vi "Save_Data_file_header_and_path_configuration.vi"(1 "Save":bool, 2 "path":path, 3 "File name":string="Name") -> (0 "Output Path":path)   [LabVIEW 2018]
uses:
  <vilib>/Utility/file.llb/Write To Spreadsheet File (string).vi
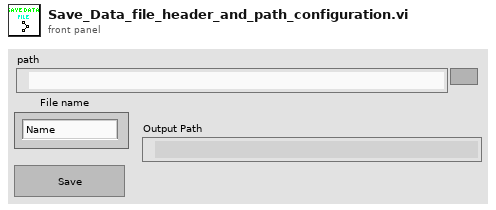
[diagram p1: front panel]
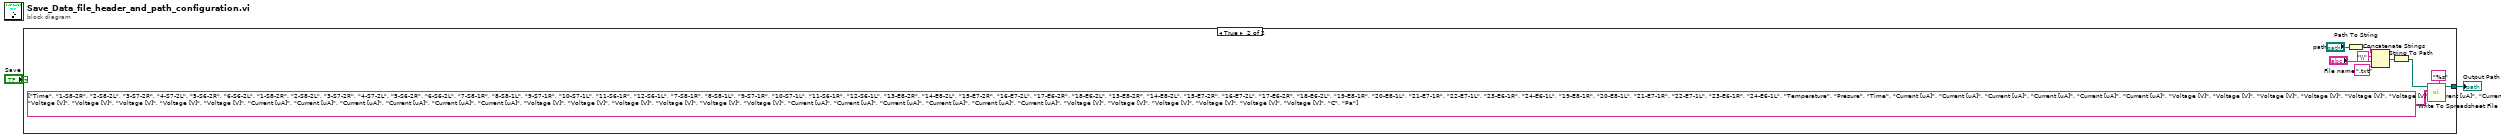
[diagram p0: block diagram]
diagram:
  n1 = case shown="True" "Save" {
    tunnel: [_ w6] -> w1
    frame False {
    }
    frame True {
      n2 = Path To String(path="path") -> (string=w5:string)
      n3 = Concatenate Strings(w5, "\\" ("string"), "File name", ".txt" ("string")) -> (w11:string)
      n4 = String To Path(string=w11) -> (path=w12:path)
      n5 = call-poly <vilib>:"Write To Spreadsheet File.vi"("format (%s)"="%s", "2D data"=string[][] [["Time", "1-S8-2R", "2-S8-2L", "3-S7-2R", "4-S7-2L", "5-S6-2R", "6-S6-2L", "1-S8-2R", "2-S8-2L", "3-S7-2R", "4-S7-2L", "5-S6-2R", "6-S6-2L", "7-S8-1R", "8-S8-1L", "9-S7-1R", "10-S7-1L", "11-S6-1R", "12-S6-1L", "7-S8-1R", "8-S8-1L", "9-S7-1R", "10-S7-1L", "11-S6-1R", "12-S6-1L", "13-E8-2R", "14-E8-2L", "15-E7-2R", "16-E7-2L", "17-E6-2R", "18-E6-2L", "13-E8-2R", "14-E8-2L", "15-E7-2R", "16-E7-2L", "17-E6-2R", "18-E6-2L", "19-E8-1R", "20-E8-1L", "21-E7-1R", "22-E7-1L", "23-E6-1R", "24-E6-1L", "19-E8-1R", "20-E8-1L", "21-E7-1R", "22-E7-1L", "23-E6-1R", "24-E6-1L", "Temperature", "Presure"], ["Time", "Current [uA]", "Current [uA]", "Current [uA]", "Current [uA]", "Current [uA]", "Current [uA]", "Voltage [V]", "Voltage [V]", "Voltage [V]", "Voltage [V]", "Voltage [V]", "Voltage [V]", "Current [uA]", "Current [uA]", "Current [uA]", "Current [uA]", "Current [uA]", "Current [uA]", "Voltage [V]", "Voltage [V]", "Voltage [V]", "Voltage [V]", "Voltage [V]", "Voltage [V]", "Current [uA]", "Current [uA]", "Current [uA]", "Current [uA]", "Current [uA]", "Current [uA]", "Voltage [V]", "Voltage [V]", "Voltage [V]", "Voltage [V]", "Voltage [V]", "Voltage [V]", "Current [uA]", "Current [uA]", "Current [uA]", "Current [uA]", "Current [uA]", "Current [uA]", "Voltage [V]", "Voltage [V]", "Voltage [V]", "Voltage [V]", "Voltage [V]", "Voltage [V]", "C", "Pa"]], "file path (dialog if empty)"=w12) -> ("new file path (Not A Path if cancelled)"=w6:path)  [unwired: 5 in]
    }
  }
  "Output Path" <- w1
